vi "Revision Query.vi"(0 "VISA resource name":refnum<visa-resource-name>, 1 "Check For SCPI Errors? (T)":bool=TRUE, 11 "error in (no error)":errorcluster) -> (4 "VISA resource name out":refnum<visa-resource-name>, 8 "Instrument Driver Revision":string, 10 "Instrument Firmware Revision":string, 15 "error out":errorcluster)   [LabVIEW 2009, in "Keithley 6514 LV 2009.lvlib"]
doc: "Queries the current instrument firmware revision and instrument driver revision."
uses:
  Keithley 6514 LV 2009.lvlib
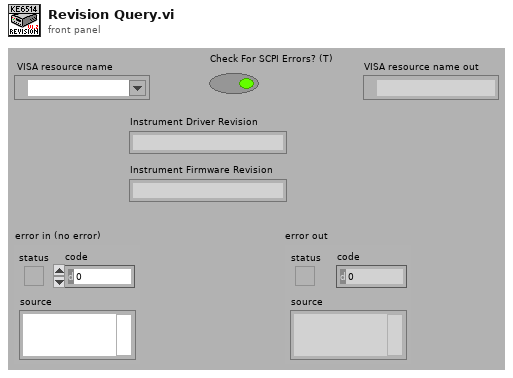
[diagram p1: front panel]
types:
  T1 = enum32{"invalid app kind", "Development System", "Run Time System", "Student Edition", "Embedded LabVIEW", "Evaluation", "Custom"}
  T2 = cluster{"Major":u16, "Minor":u16, "Fix":u16, "Build":u16}
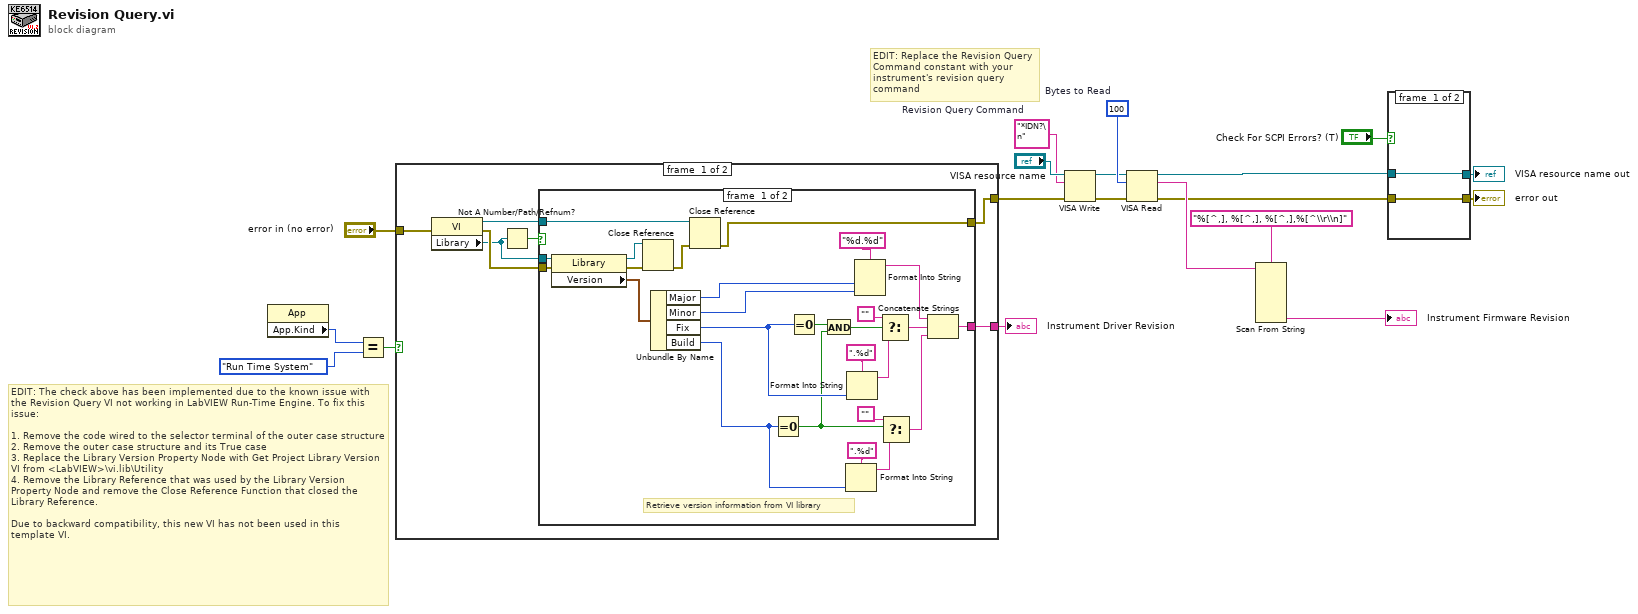
[diagram p0: block diagram]
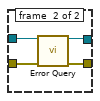
[diagram p2: hidden frame]
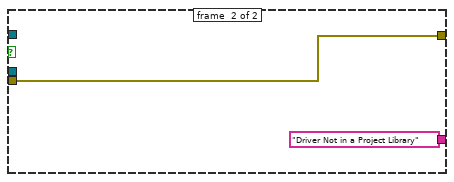
[diagram p3: hidden frame]
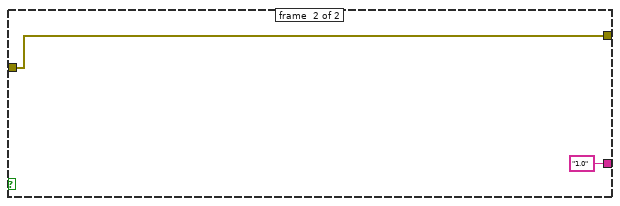
[diagram p4: hidden frame]
diagram:
  w14 = "*IDN?\n"  # Revision Query Command
  w17 = u32 100  # Bytes to Read
  # "EDIT: The check above has been implemented due to the known issue with the Revision Query VI not working in LabVIEW Run-Time Engine. To fix this issue:\n\n1. Remove the code wired to the selector terminal of the outer case structure\n2. Remove the outer case structure and its True case\n3. Replace the Library Version Property Node with Get Project Library Version VI from <LabVIEW>\\vi.lib\\Utility\n4. Remove the Library Reference that was used by the Library Version Property Node and remove the Close Reference Function that closed the Library Reference.\n\nDue to backward compatibility, this new VI has not been used in this template VI."
  # "EDIT: Replace the Revision Query\nCommand constant with your\ninstrument's revision query\ncommand"
  n1 = property class="App"() -> ("App.Kind"=w3:T1)  [unwired: 2 in, 2 out]
  n2 = Equal?(x=w3, y=T1."Run Time System" ("Application:Kind")) -> (x = y?=w4:bool)
  n3 = case shown="False" w4 {
    tunnel: [w22 "1.0"] -> w7
    tunnel: "error in (no error)" -> [w21 w55]
    tunnel: [w20 w55] -> w5
    frame #0 {
      n4 = property class="VI"(error in=w21) -> (reference out=w26:refnum<vi>, error out=w25:errorcluster, "Library"=w24:refnum<vi>)  [unwired: 1 in]
      n5 = Not A Number/Path/Refnum?(number/path/refnum=w24) -> (NaN/Path/Refnum?=w23:bool)
      n6 = case shown="False" w23 {
        tunnel: w26 -> [w49 _]
        tunnel: w25 -> [w34 w54]
        tunnel: [w29 w54] -> w20
        tunnel: [w28 "Driver Not in a Project Library"] -> w22
        tunnel: w24 -> [w27 _]
        frame #0 {
          # "Retrieve version information from VI library"
          n7 = property class="Library"(reference=w27, error in=w34) -> (reference out=w51:refnum<vi>, error out=w52:errorcluster, "Version"=w48:T2)
          n8 = Close Reference(reference=w51, error in (no error)=w52) -> (error out=w50:errorcluster)
          n9 = Unbundle By Name(w48) -> ("Major"=w37:u16, "Minor"=w36:u16, "Fix"=w33:u16, "Build"=w35:u16)
          n10 = Close Reference(reference=w49, error in (no error)=w50) -> (error out=w29:errorcluster)
          n11 = Equal To 0?(x=w35) -> (x = 0?=w31:bool)
          n12 = Equal To 0?(x=w33) -> (x = 0?=w32:bool)
          n13 = And(x=w32, y=w31) -> (x .and. y?=w30:bool)
          n14 = Format Into String(format string=".%d", w35) -> (resulting string=w41:string)  [unwired: 2 in, 1 out]
          n15 = Format Into String(format string=".%d", w33) -> (resulting string=w45:string)  [unwired: 2 in, 1 out]
          n16 = Format Into String(format string="%d.%d", w37, w36) -> (resulting string=w43:string)  [unwired: 2 in, 1 out]
          n17 = Select(t="", s=w30, f=w45) -> (s? t:f=w42:string)
          n18 = Select(t="", s=w31, f=w41) -> (s? t:f=w38:string)
          n19 = Concatenate Strings(w43, w42, w38) -> (w28:string)
        }
        frame #1 {
        }
      }
    }
    frame #1 {
    }
  }
  "Instrument Driver Revision" <- w7
  n20 = VISA Write(VISA resource name="VISA resource name", write buffer=w14, error in (no error)=w5) -> (VISA resource name out=w16:refnum<visa-resource-name>, error out=w15:errorcluster)  [unwired: 1 out]
  n21 = VISA Read(VISA resource name=w16, byte count=w17, error in (no error)=w15) -> (VISA resource name out=w10:refnum<visa-resource-name>, read buffer=w13:string, error out=w11:errorcluster)  [unwired: 1 out]
  n22 = Scan From String(format string="%[^,], %[^,], %[^,],%[^\\r\\n]", input string=w13) -> (output 4=→"Instrument Firmware Revision":string)  [unwired: 9 in, 3 out]
  n23 = case shown="False" "Check For SCPI Errors? (T)" {
    tunnel: w11 -> [w57 w62]
    tunnel: w10 -> [w58 w61]
    tunnel: [w58 w60] -> w9
    tunnel: [w57 w59] -> w8
    frame #0 {
    }
    frame #1 {
      n24 = call "Error Query.vi"("VISA Resource In"=w61, "error in (no error)"=w62) -> ("VISA Resource Out (dupl)"=w60:refnum<visa-resource-name>, "error out"=w59:errorcluster)  [unwired: 10 in, 2 out]
    }
  }
  "VISA resource name out" <- w9
  "error out" <- w8
